vi "ReadRobotFile.vi"() -> ()   [LabVIEW 2014]
uses:
  <vilib>/Utility/file.llb/Read From Spreadsheet File (string).vi
panel:
  out "all rows 2":string[](array[string])
  out "all rows":string[][](array[string])
  in  "Path":path
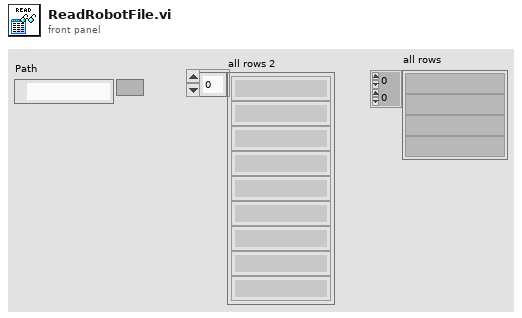
[diagram p1: front panel]
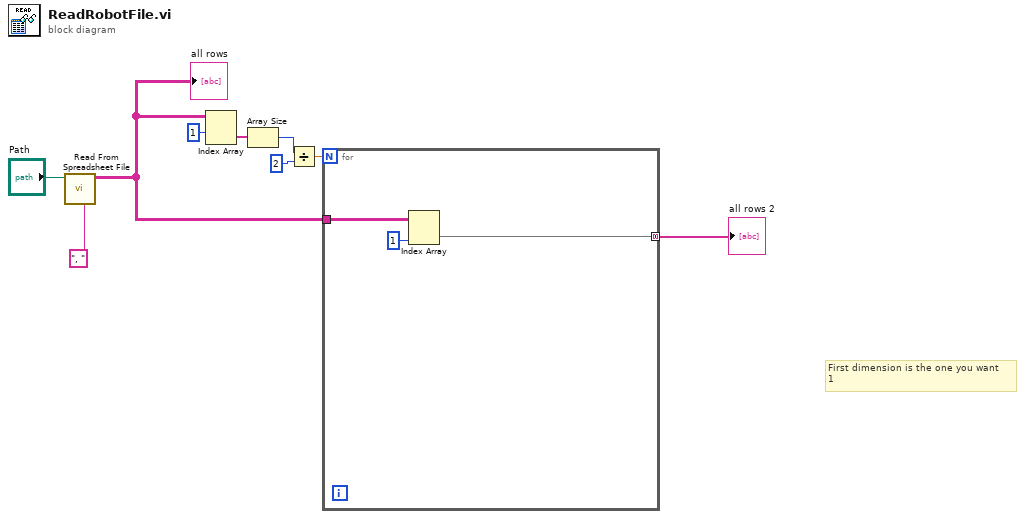
[diagram p0: block diagram]
diagram:
  # "First dimension is the one you want\n1"
  n1 = call-poly <vilib>:"Read From Spreadsheet File.vi"("delimiter (\\t)"=", " ("delimiter (\\t)"), "file path (dialog if empty)"="Path") -> ("all rows"=w5:string[][])  [unwired: 5 in, 4 out]
  "all rows" <- w5
  n2 = Index Array(array=w5, index (row)=1 ("index")) -> (element=w4:string[])  [unwired: 1 in]
  n3 = Array Size(array=w4) -> (size(s)=w2:i32)
  n4 = Divide(x=w2, y=2) -> (x/y=w1:dbl)
  n5 = for {
    N: w1 -> [_]
    tunnel: w5 -> [w12]
    tunnel: [w11] -> w7 mode=concatenating
    n6 = Index Array(array=w12, index (col)=1 ("disabled index (col)")) -> (element=w11:string[])  [unwired: 1 in]
  }
  "all rows 2" <- w7
